vi "PmodGYROOpen.vi"(7 "I2C Channel (0)":u8, 8 "error in (no error)":errorcluster, 9 "Resolution (dps)":enum16{"2000", "500", "250"}(ring), 10 "Address":enum8{"0x68", "0x69"}(ring)=enum."0x69") -> (0 "error out":errorcluster, 1 "Resolution (dps)":enum16{"2000", "500", "250"}(ring))   [LabVIEW 2018]
doc: "Open I2C communication.\n\nWrite 0xF to register 0x20 to power on PmodGYRO\n\nWrite different values to register 0x23 to configure the resolution of PmodGYRO"
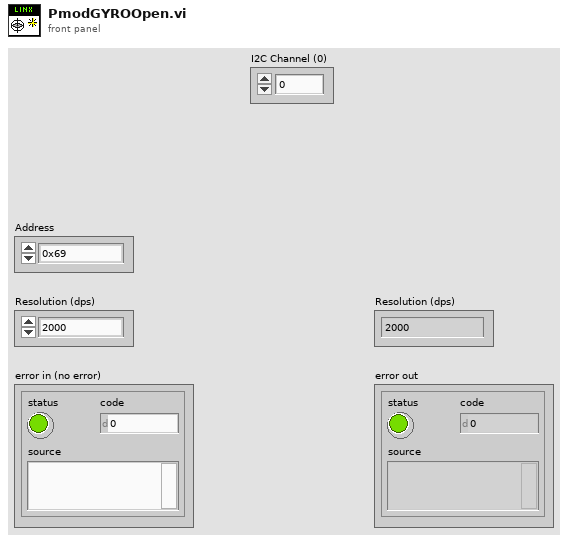
[diagram p1: front panel]
types:
  T1 = typedef "WPI_I2CDevRef.ctl" = cluster{"DevStatus":errorcluster, "Device Address":u8, "Handle":i32, "I2C Bus":T2}
  T2 = typedef "i2c_bus.ctl" = enum16{"I2C On-Board", "I2C MXP", "Invalid"}
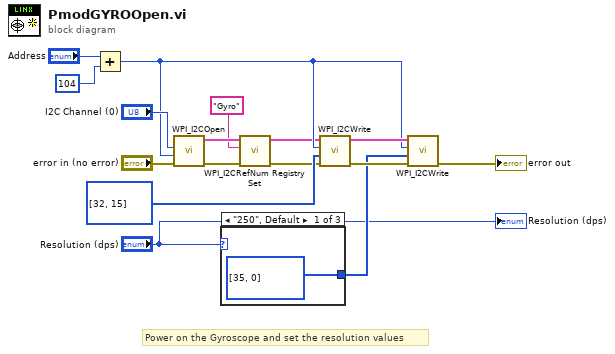
[diagram p0: block diagram]
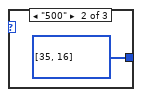
[diagram p2: hidden frame]
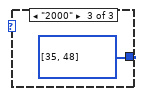
[diagram p3: hidden frame]
diagram:
  # "Power on the Gyroscope and set the resolution values"
  n1 = Add(x="Address", y=u8 104) -> (x+y=w6:u8)
  n2 = call <vilib>:"WPI_I2COpen.vi"("error in"="error in (no error)", "Device Address"=w6, "I2C Bus"="I2C Channel (0)") -> ("error out"=w3:errorcluster, "I2CDevRef"=w5:T1)  [unwired: 7 in]
  n3 = case shown="\"250\", Default" "Resolution (dps)" {
    tunnel: [u8[] [35, 0] ("Data") u8[] [35, 16] ("Data") u8[] [35, 48] ("Data")] -> w13
    frame "250", Default {
    }
    frame "500" {
    }
    frame "2000" {
    }
  }
  n4 = call <vilib>:"WPI_I2CRefNum Registry Set.vi"("error in (no error)"=w3, "refnum name"="Gyro", "I2CDevRef"=w5) -> ("error out"=w2:errorcluster, "I2CDevRef"=w4:T1)  [unwired: 7 in]
  n5 = call <vilib>:"WPI_I2CWrite.vi"("error in (no error)"=w2, "I2CDataToSend"=u8[] [32, 15] ("Data"), "I2CRegister"=w6, "I2CDevRef"=w4) -> ("error out"=w14:errorcluster, "I2CDevRef"=w16:T1)  [unwired: 6 in]
  n6 = call <vilib>:"WPI_I2CWrite.vi"("error in (no error)"=w14, "I2CDataToSend"=w13, "I2CRegister"=w6, "I2CDevRef"=w16) -> ("error out"=→"error out":errorcluster)  [unwired: 6 in, 1 out]
  "Resolution (dps)" <- "Resolution (dps)"
